vi "LET Output v2.vi"() -> ()   [LabVIEW 2010]
doc: "Cont(inuous) Acq(uire) & Chart (hw timed) demonstrates the hardware timed, non-buffered technique of data acquisition. The scan clock on the board controls acquisition timing. Acquired scans are read directly from the device's FIFO using AI Single Scan. \n\nThe acquisition is configured with no buffer, and the on-board scan clock started at the selected scan rate. In the first loop iteration, the newest (most recent) scan is read from the FIFO. In each subsequent loop iteration AI Single Scan is called to read the oldest scan from the FIFO. Then if a scan is missed because the acquisition does not keep up, an error message will be displayed, and the acquisition stopped. Each scan is plotted on the chart after it is read. \n\nA common reason to use non-buffered acquisition is that some kind of processing needs to be done for each data point. You will probably want to add more functions to the diagram to customize this VI for your application. The acquisition rate you can achieve depends on how much processing and display the VI must do. This VI calls a subVI named My Single-Scan Processing. Add whatever processing you need to this subVI, or replace it with one of your own. The data processing subVI also demonstrates how to use error clusters in your own subVIs, so they can be included in the error data flow chain.\n\nBefore running this VI, set the values of the controls on the front panel. Select Show Help Window from the Help menu to see a description of each control. If the values you select for all the controls are values you will usually use, select Make Current Values Default from the Operate menu and save the VI. Or, you may save individual control's default values by popping up on the control, selecting Data Operations, then selecting Make Current Value Default, and saving the VI."
uses:
  <instrlib>/agilent_b2900_series/Agilent B2900 Series/Public/Configure/Measurement/Configure Measurement (Current).vi
  <instrlib>/agilent_b2900_series/Agilent B2900 Series/Public/Configure/Measurement/Configure Measurement (Voltage).vi
  <vilib>/Analysis/Matrix/Numeric/Conversions/Matrix To Array - RM.vi
  <vilib>/Utility/file.llb/Write To Spreadsheet File (DBL).vi
  <instrlib>/agilent_b2900_series/Agilent B2900 Series/Agilent B2900 Series.lvlib
  <vilib>/Analysis/Matrix/NI_Matrix.lvlib
panel:
  out "Real 2D Array":dbl[][](array[numeric])
  out "data matrix":dbl[][](array[numeric])
  out "Igs array 2":dbl[][](array[numeric])
  out "Vgs array 2":dbl[][](array[numeric])
  out "Vds array 2":dbl[][](array[numeric])
  out "Corrected PD current array 2":dbl[][](array[numeric])
  out "Ids array 2":dbl[][](array[numeric])
  out "corrected PD current array":dbl[](array[numeric])
  out "Vds array":dbl[](array[numeric])
  out "Ids array":dbl[](array[numeric])
  out "Vgs array":dbl[](array[numeric])
  out "Igs array":dbl[](array[numeric])
  in  "Tab Control":T1(tab)
  in  "keithley address":string="GPIB0::20::INSTR"
  in  "agilent address":refnum<visa-resource-name>="GPIB0::23::INSTR"
  in  "Initial Vds (V)\n(100 scans/sec)":sgl caption="Initial Vds (V)" format="%.2f"
  in  "Vds step (V)":sgl=1.0 format="%.2f"
  in  "Vds delay time":sgl=10.0 caption="Vds delay time (ms)" format="%.2f"
  in  "Vds delay after first value (ms)":sgl=10.0 format="%.2f"
  in  "Final Vds(V)":sgl=60.0 format="%.2f"
  in  "light emission ON/OFF":bool=TRUE
  in  "Vgs step (V)":sgl=20.0 format="%.2f"
  in  "Final Vgs (V)":sgl=60.0 format="%.2f"
  in  "Initial Vgs (V)":sgl format="%.2f"
  in  "Vgs hold time (ms)":i32=10
  in  "Compliance Voltage (channel 2)":dbl=60.0
  in  "Compliance Current (channel 1)":dbl=0.001
  in  "Compliance Voltage (channel 1)":dbl=60.0
  in  "Compliance Current (channel 2)":dbl=0.0001
  in  "keithley compliance limit":dbl(ring)=0.025 items=["25uA"=2.5e-05, "250uA"=0.00025, "2.5mA"=0.0025, "25mA"=0.025]
  in  "Loop":bool=TRUE
  in  "keithley current resolution":dbl=0.0001 format="%^.2e"
  in  "Current Auto Range Mode (0: Normal)":i32(ring) items=["Normal", "Resolution", "Speed"]
  in  "Voltage Auto Range Mode (0: Normal)":i32(ring) items=["Normal", "Resolution", "Speed"]
  in  "aperture time":dbl(ring)=-2.0 format="%.2f" items=["KE6485_VAL_RATE_FAST"=-1.0, "KE6485_VAL_RATE_MEDIUM"=-2.0, "KE6485_VAL_RATE_SLOW"=-3.0]
  in  "Auto Current NPLC (F: Disable)":bool
  in  "Current NPLC (0.1)":dbl=0.1
  in  "Auto Voltage NPLC(F: Disable)":bool
  in  "Voltage NPLC (0.1 PLC)":dbl=0.1
  out "Current Scan":cluster{dbl[], dbl[]}(graph)
  out "Applied Vds":sgl caption="current VDS (V)" format="%.2f"
  out "Applied Vgs":sgl caption="current VDS (V)" format="%.2f"
  out "Measured Ids":dbl format="%.2e"
  out "Measured Vds":dbl
  out "corrected PD current":dbl format="%^.2e"
  out "dark PD current (A)":dbl format="%^.2e"
  out "PD current":dbl format="%^.2e"
  out "Measured Igs":dbl
  out "Measured Vgs":dbl
  out "channel 2 status":bool
  out "channel 1 status":bool
  out "Current Scan 2":cluster{dbl[], dbl[]}(graph) caption="Current Scan"
  out "half  points":sgl
  out "Vds points":sgl
  out "Vgs points":sgl
  out "?":cluster{dbl[], dbl[]}[](graph)
  out "?":cluster{dbl[], dbl[]}[](graph)
  in  "error in keithley":errorcluster
  out "keithley address out":refnum<k15>
  out "error out keithley":errorcluster
  out "error out agilent":errorcluster
  out "Agilent address out":refnum<visa-resource-name>
  # "FET output v2"
  # "Drain-Source Setting"
  # "Gate Setting"
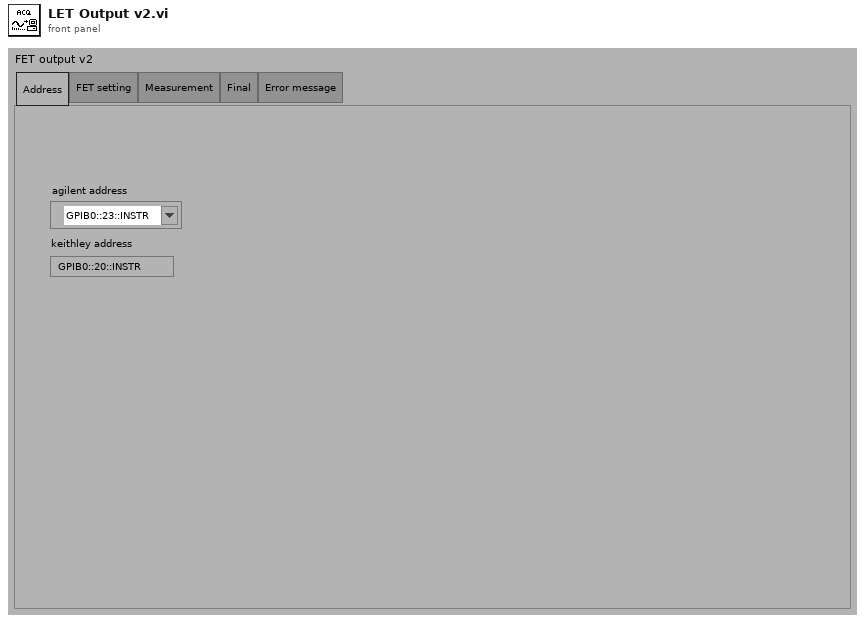
[diagram p1: front panel]
types:
  T1 = enum32{"Address", "FET setting", "Measurement", "Final", "Error message"}
  T2 = typedef "NI_Matrix.lvlib/RealMatrix.ctl" = dbl[][]
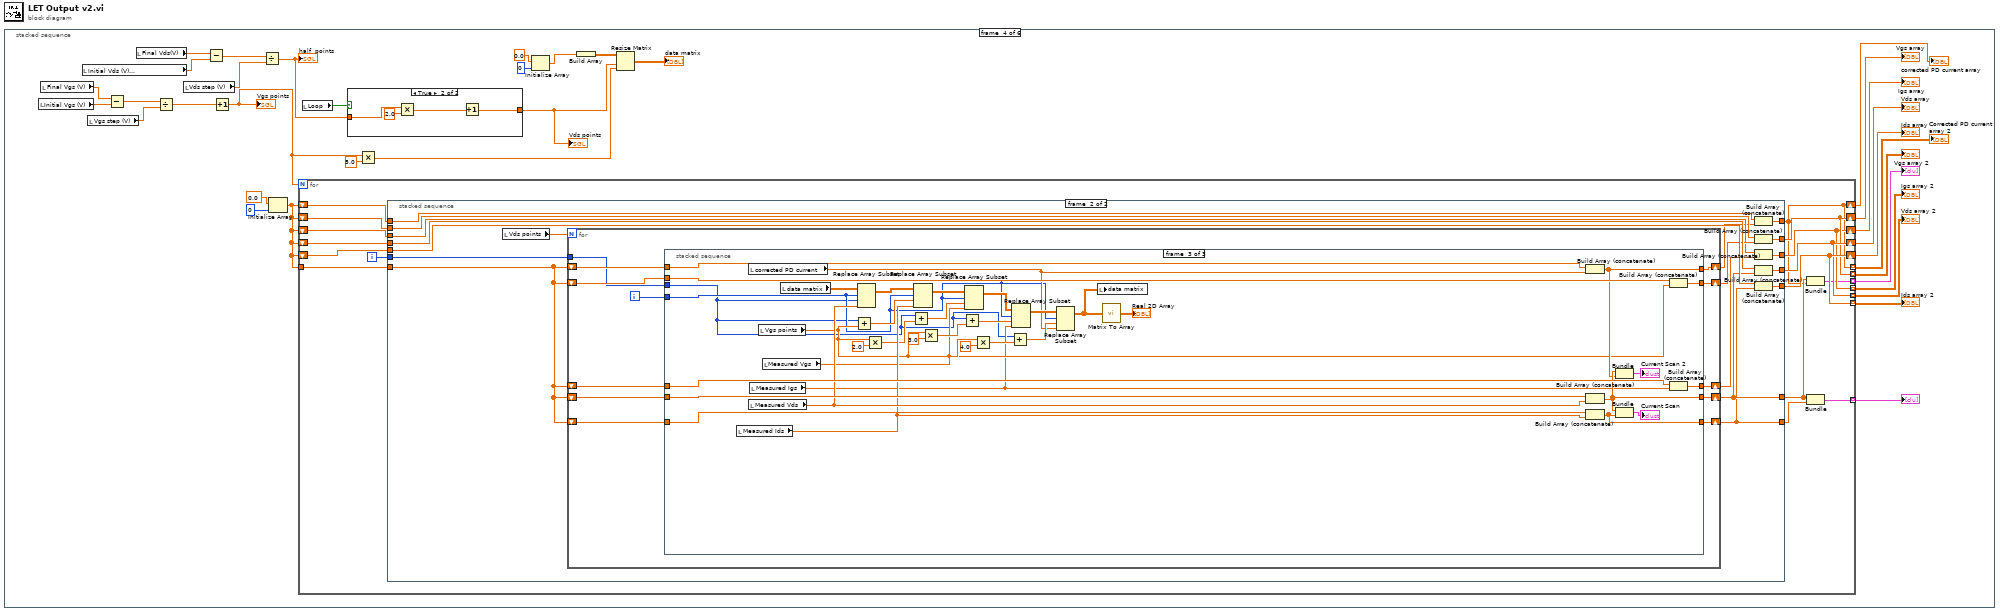
[diagram p0: block diagram]
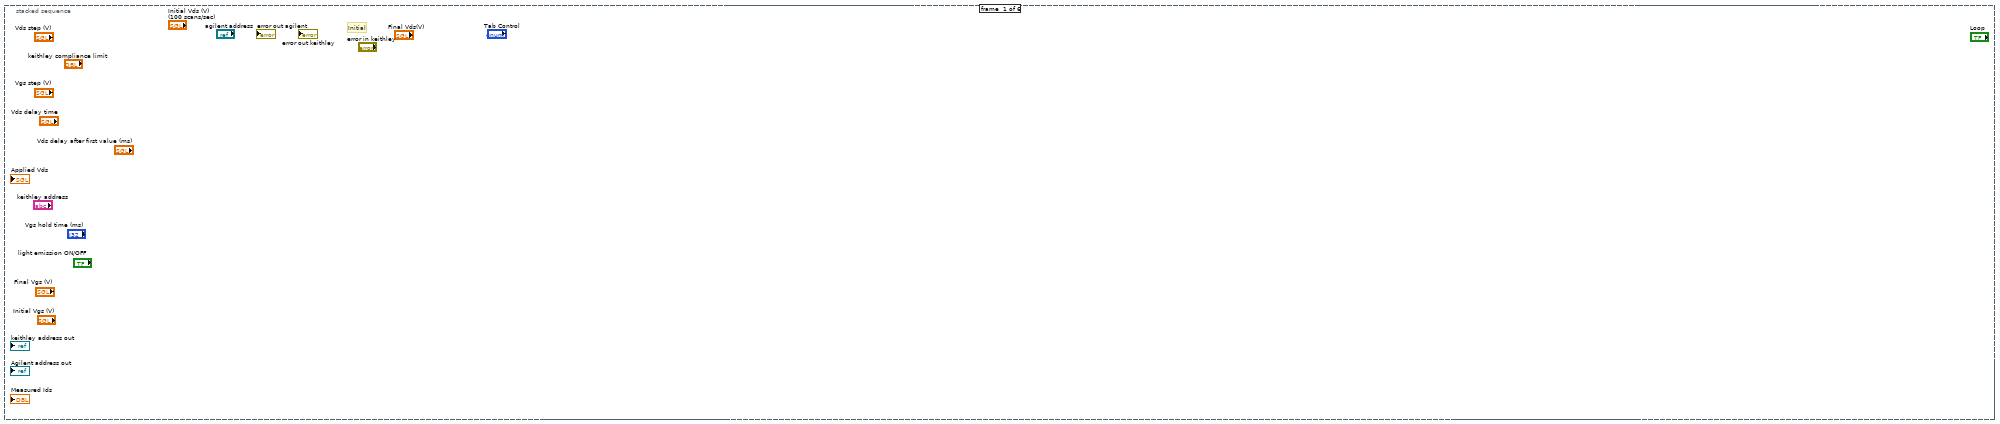
[diagram p2: hidden frame]
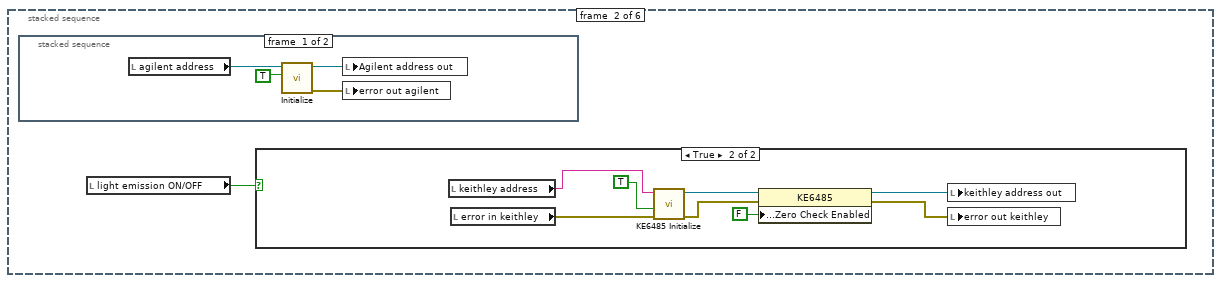
[diagram p3: hidden frame]
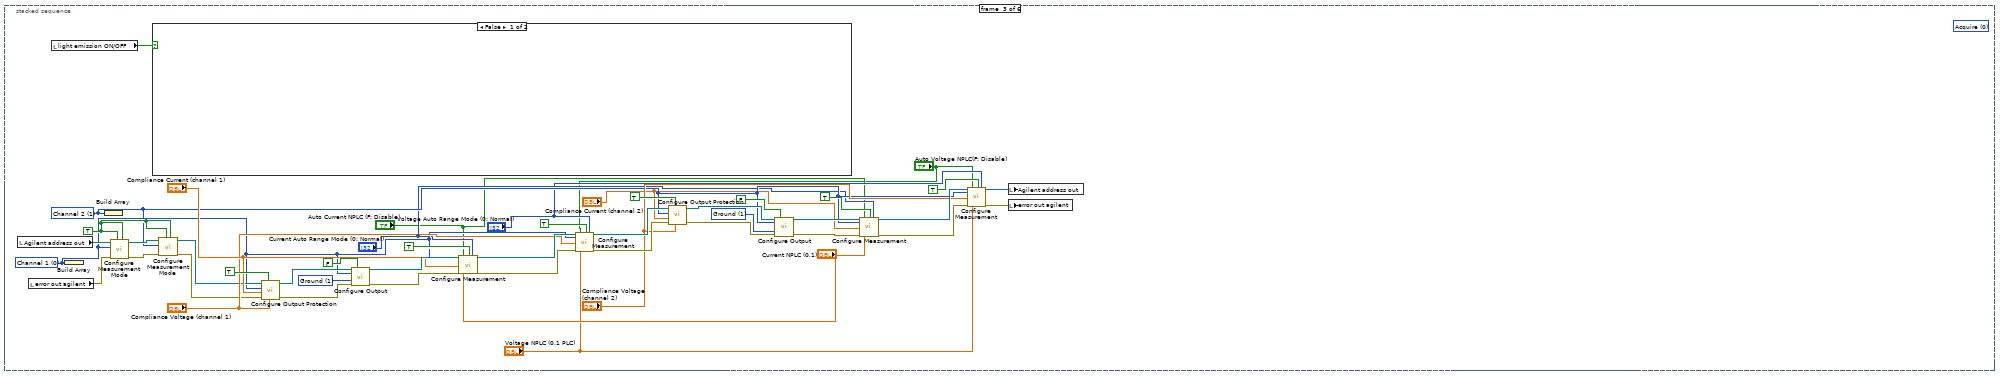
[diagram p6: hidden frame]
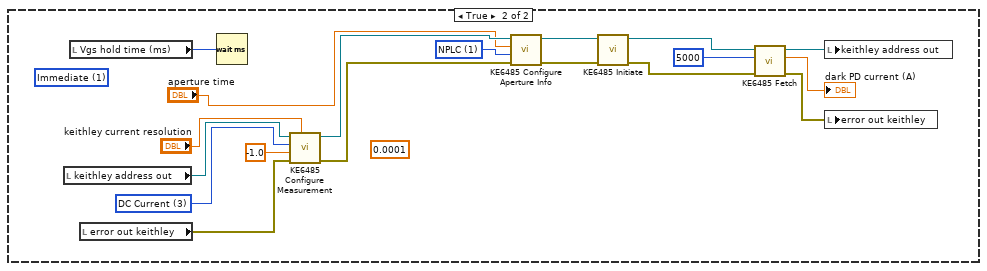
[diagram p7: hidden frame]
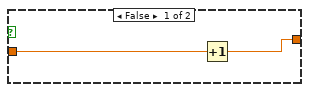
[diagram p8: hidden frame]
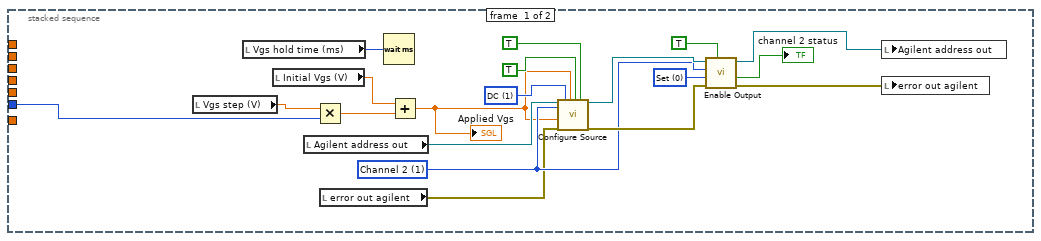
[diagram p9: hidden frame]
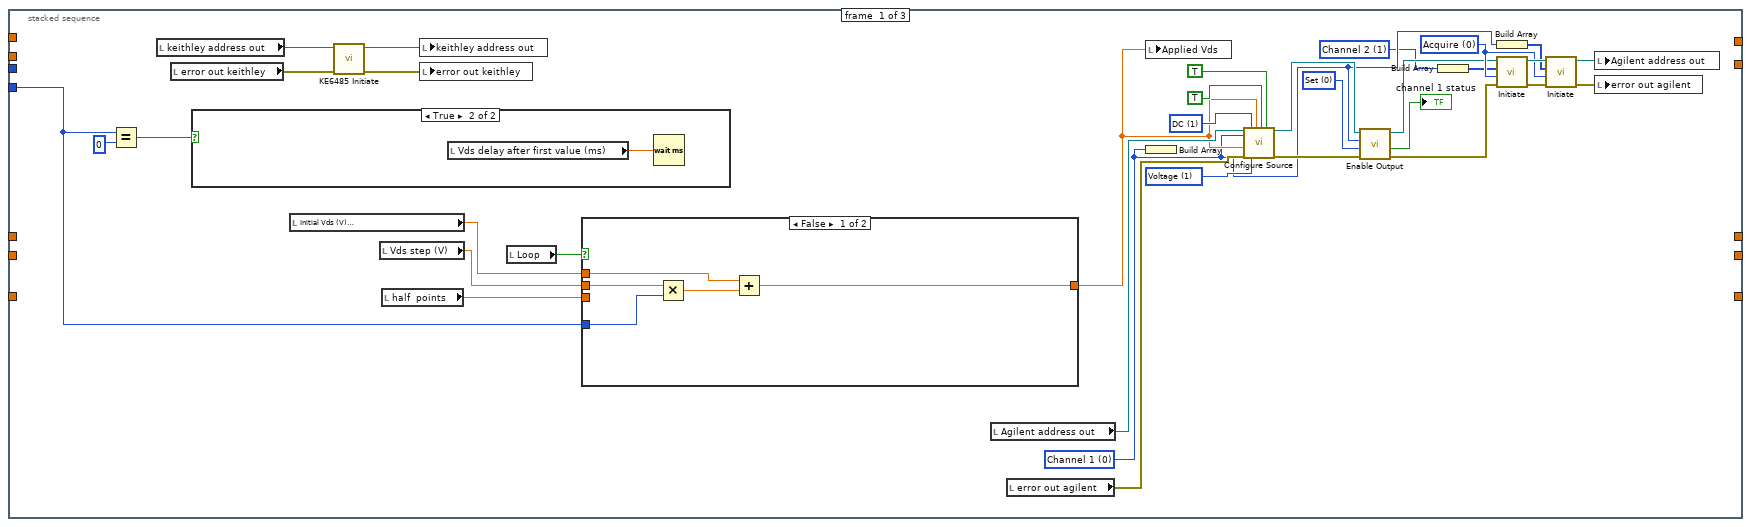
[diagram p10: hidden frame]
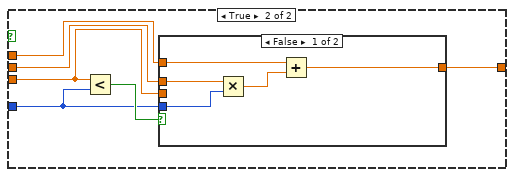
[diagram p11: hidden frame]
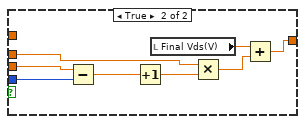
[diagram p12: hidden frame]
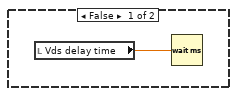
[diagram p13: hidden frame]
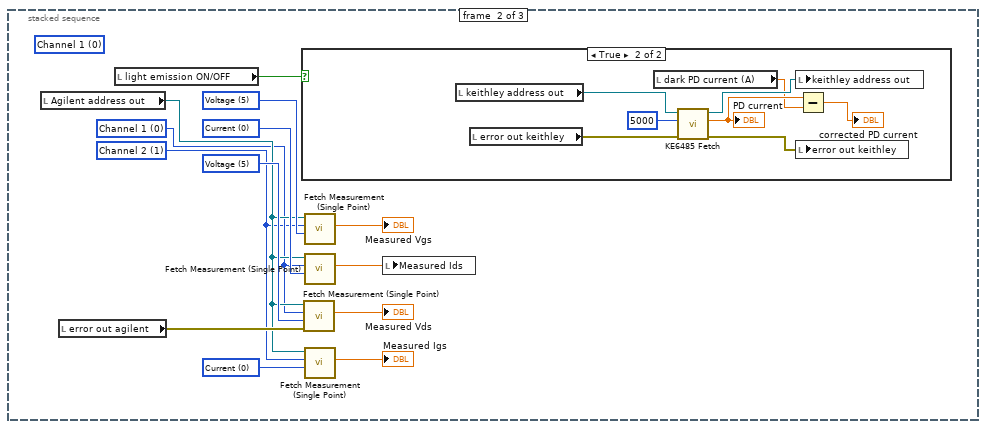
[diagram p14: hidden frame]
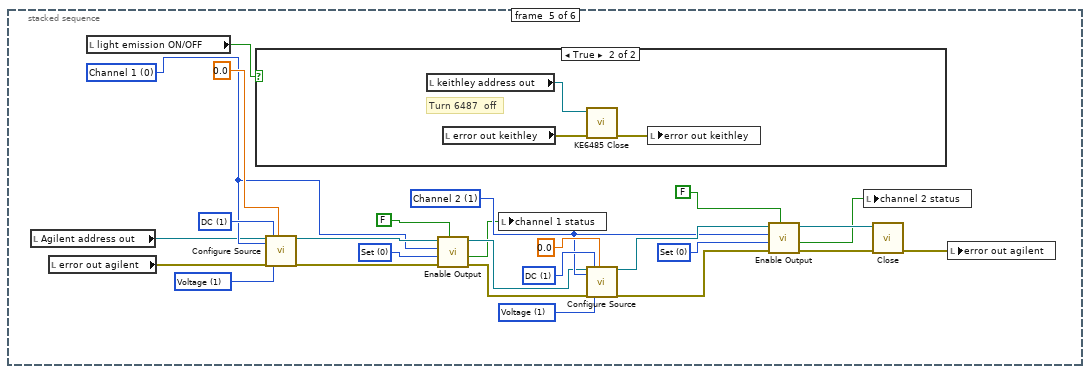
[diagram p16: hidden frame]
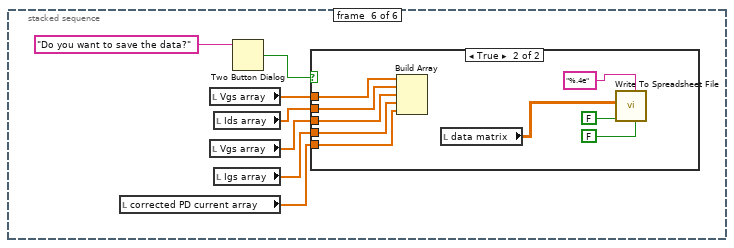
[diagram p18: hidden frame]
diagram:
  n1 = stacked-sequence {
    frame #0 {
      # "Initial"
    }
    frame #1 {
      n2 = stacked-sequence {
        frame #0 {
          n3 = local read "agilent address"() -> (w2:refnum<visa-resource-name>)
          n4 = call <instrlib>:"Initialize.vi"("ID Query (True)"=TRUE, "VISA resource name"=w2) -> ("error out"=w3:errorcluster, "VISA resource name out"=w4:refnum<visa-resource-name>)  [unwired: 8 in]
          n5 = local write "Agilent address out"(w4) -> ()
          n6 = local write "error out agilent"(w3) -> ()
        }
        frame #1 {
        }
      }
      n7 = local read "light emission ON/OFF"() -> (w1:bool)
      n8 = case shown="True" w1 {
        frame False {
        }
        frame True {
          n9 = local read "keithley address"() -> (w12:string)
          n10 = local read "error in keithley"() -> (w13:errorcluster)
          n11 = call <instrlib>:"KE6485 Initialize.vi"("error in (no error)"=w13, "reset device"=TRUE, "resource name"=w12) -> ("error out"=w10:errorcluster, "instrument handle out"=w9:refnum<k15>)  [unwired: 1 in, 6 out]
          n12 = property class="KE6485"(reference=w9, error in=w10, "System Settings:Zero Check Enabled"=FALSE) -> (reference out=w8:refnum<k15>, error out=w7:errorcluster)
          n13 = local write "keithley address out"(w8) -> ()
          n14 = local write "error out keithley"(w7) -> ()
        }
      }
    }
    frame #2 {
      (unwired) 0 items=["Acquire", "Transient", "Both"] ("Device Action (2: Both)")
      w30 = TRUE ("Enable Voltage Measurement (T: Enable)")
      w42 = 1 items=["Float", "Ground"] ("Low Terminal State (1: Ground)")
      w22 = 1 items=["Channel 1", "Channel 2"] ("Channel (0: Channel 1)")
      w52 = 1 items=["Float", "Ground"] ("Low Terminal State (1: Ground)")
      w23 = 0 items=["Channel 1", "Channel 2"] ("Channel (0: Channel 1)")
      n15 = local read "Agilent address out"() -> (w25:refnum<visa-resource-name>)
      n16 = local read "error out agilent"() -> (w27:errorcluster)
      n17 = local read "light emission ON/OFF"() -> (w59:bool)
      n18 = Build Array(w23) -> ()  [unwired: 1 out]
      n19 = Build Array(w22) -> ()  [unwired: 1 out]
      n20 = call <instrlib>:"Configure Measurement Mode.vi"("Enable Current Measurement (T: Enable)"=w30, "Enable Voltage Measurement (T: Enable)"=w30, "error in (no error)"=w27, "Channel (0: Channel 1)"=w23, "VISA resource name"=w25) -> ("error out"=w28:errorcluster, "VISA resource name out"=w29:refnum<visa-resource-name>)  [unwired: 5 in]
      n21 = case shown="False" w59 {
        frame False {
        }
        frame True {
          w65 = 1 items=["NPLC"=1] ("aperture time unit")
          (unwired) 0.0001 ("resolution (absolute)")
          (unwired) 1 items=["Immediate"=1, "Interval"=10, "Trigger Link 1"=1001, "Trigger Link 2"=1002, "Trigger Link 3"=1003, "Trigger Link 4"=1004, "Trigger Link 5"=1005, "Trigger Link 6"=1006] ("sample trigger")
          w75 = 3 items=["DC Volts"=1, "DC Current"=3, "2 Wire Resistance"=5, "Charge"=1004] ("measurement function")
          n22 = local read "keithley address out"() -> (w70:refnum<k15>)
          n23 = local read "Vgs hold time (ms)"() -> (w77:i32)
          n24 = local read "error out keithley"() -> (w69:errorcluster)
          n25 = Wait (ms)(milliseconds to wait=w77) -> ()  [unwired: 1 out]
          n26 = call <instrlib>:"KE6485 Configure Measurement.vi"("resolution (absolute)"="keithley current resolution", "error in (no error)"=w69, "range"=-1.0, "measurement function"=w75, "instrument handle"=w70) -> ("error out"=w64:errorcluster, "instrument handle out"=w63:refnum<k15>)  [unwired: 5 in]
          n27 = call <instrlib>:"KE6485 Configure Aperture Info.vi"("error in (no error)"=w64, "aperture time unit"=w65, "aperture time"="aperture time", "instrument handle"=w63) -> ("error out"=w61:errorcluster, "instrument handle out"=w62:refnum<k15>)  [unwired: 6 in]
          n28 = call <instrlib>:"KE6485 Initiate.vi"("error in (no error)"=w61, "instrument handle"=w62) -> ("error out"=w67:errorcluster, "instrument handle out"=w68:refnum<k15>)  [unwired: 8 in]
          n29 = call <instrlib>:"KE6485 Fetch.vi"("error in (no error)"=w67, "maximum time (ms)"=5000, "instrument handle"=w68) -> ("error out"=w72:errorcluster, "reading"=→"dark PD current (A)":dbl, "instrument handle out"=w71:refnum<k15>)  [unwired: 6 in]
          n30 = local write "keithley address out"(w71) -> ()
          n31 = local write "error out keithley"(w72) -> ()
        }
      }
      n32 = call <instrlib>:"Configure Measurement Mode.vi"("Enable Current Measurement (T: Enable)"=w30, "Enable Voltage Measurement (T: Enable)"=w30, "error in (no error)"=w28, "Channel (0: Channel 1)"=w22, "VISA resource name"=w29) -> ("error out"=w26:errorcluster, "VISA resource name out"=w24:refnum<visa-resource-name>)  [unwired: 5 in]
      n33 = call <instrlib>:"Configure Output Protection.vi"("Compliance Voltage (2 V)"="Compliance Voltage (channel 1)", "Enable Output Protection (T: Enable)"=TRUE, "error in (no error)"=w26, "Compliance Current (0.0001 A)"="Compliance Current (channel 1)", "Channel (0: Channel 1)"=w23, "VISA resource name"=w24) -> ("error out"=w54:errorcluster, "VISA resource name out"=w53:refnum<visa-resource-name>)  [unwired: 4 in]
      n34 = call <instrlib>:"Configure Output.vi"("VISA resource name"=w53, "Auto Output-Off (F: Disable)"=FALSE, "Channel (0: Channel 1)"=w23, "Low Terminal State (1: Ground)"=w52, "error in (no error)"=w54) -> ("VISA resource name out"=w50:refnum<visa-resource-name>, "error out"=w51:errorcluster)  [unwired: 9 in]
      n35 = call-poly <instrlib>:"Configure Measurement.vi"("VISA resource name"=w50, "Channel (0: Channel 1)"=w23, "Current Range (0.0001 A)"="Compliance Current (channel 1)", "error in (no error)"=w51, "Auto Current NPLC (F: Disable)"="Auto Current NPLC (F: Disable)", "Current NPLC (0.1)"="Current NPLC (0.1)", "Current Auto Range (T: Enable)"=TRUE, "Current Auto Range Mode (0: Normal)"="Current Auto Range Mode (0: Normal)") -> ("VISA resource name out"=w58:refnum<visa-resource-name>, "error out"=w57:errorcluster)  [unwired: 10 in]
      n36 = call-poly <instrlib>:"Configure Measurement.vi"("VISA resource name"=w58, "Channel (0: Channel 1)"=w23, "Voltage Range (2 V)"="Compliance Voltage (channel 1)", "error in (no error)"=w57, "Auto Voltage NPLC(F: Disable)"="Auto Voltage NPLC(F: Disable)", "Voltage NPLC (0.1 PLC)"="Voltage NPLC (0.1 PLC)", "Voltage Auto Range (T: Enable)"=TRUE, "Voltage Auto Range Mode (0: Normal)"="Voltage Auto Range Mode (0: Normal)") -> ("VISA resource name out"=w38:refnum<visa-resource-name>, "error out"=w37:errorcluster)  [unwired: 10 in]
      n37 = call <instrlib>:"Configure Output Protection.vi"("Compliance Voltage (2 V)"="Compliance Voltage (channel 2)", "Enable Output Protection (T: Enable)"=TRUE, "error in (no error)"=w37, "Compliance Current (0.0001 A)"="Compliance Current (channel 2)", "Channel (0: Channel 1)"=w22, "VISA resource name"=w38) -> ("error out"=w44:errorcluster, "VISA resource name out"=w43:refnum<visa-resource-name>)  [unwired: 4 in]
      n38 = call <instrlib>:"Configure Output.vi"("VISA resource name"=w43, "Auto Output-Off (F: Disable)"=FALSE, "Channel (0: Channel 1)"=w22, "Low Terminal State (1: Ground)"=w42, "error in (no error)"=w44) -> ("VISA resource name out"=w40:refnum<visa-resource-name>, "error out"=w41:errorcluster)  [unwired: 9 in]
      n39 = call-poly <instrlib>:"Configure Measurement.vi"("VISA resource name"=w40, "Channel (0: Channel 1)"=w22, "Current Range (0.0001 A)"="Compliance Current (channel 2)", "error in (no error)"=w41, "Auto Current NPLC (F: Disable)"="Auto Current NPLC (F: Disable)", "Current NPLC (0.1)"="Current NPLC (0.1)", "Current Auto Range (T: Enable)"=TRUE, "Current Auto Range Mode (0: Normal)"="Current Auto Range Mode (0: Normal)") -> ("VISA resource name out"=w48:refnum<visa-resource-name>, "error out"=w47:errorcluster)  [unwired: 10 in]
      n40 = call-poly <instrlib>:"Configure Measurement.vi"("VISA resource name"=w48, "Channel (0: Channel 1)"=w22, "Voltage Range (2 V)"="Compliance Voltage (channel 2)", "error in (no error)"=w47, "Auto Voltage NPLC(F: Disable)"="Auto Voltage NPLC(F: Disable)", "Voltage NPLC (0.1 PLC)"="Voltage NPLC (0.1 PLC)", "Voltage Auto Range (T: Enable)"=TRUE, "Voltage Auto Range Mode (0: Normal)"="Voltage Auto Range Mode (0: Normal)") -> ("VISA resource name out"=w21:refnum<visa-resource-name>, "error out"=w20:errorcluster)  [unwired: 10 in]
      n41 = local write "Agilent address out"(w21) -> ()
      n42 = local write "error out agilent"(w20) -> ()
    }
    frame #3 {
      n43 = local read "Initial Vgs (V)"() -> (w101:sgl)
      n44 = local read "Final Vgs (V)"() -> (w100:sgl)
      n45 = local read "Initial Vds (V)\n(100 scans/sec)"() -> (w104:sgl)
      n46 = local read "Vgs step (V)"() -> (w102:sgl)
      n47 = Subtract(x=w100, y=w101) -> (x-y=w98:sgl)
      n48 = local read "Final Vds(V)"() -> (w103:sgl)
      n49 = Divide(x=w98, y=w102) -> (x/y=w99:sgl)
      n50 = local read "Vds step (V)"() -> (w105:sgl)
      n51 = Subtract(x=w103, y=w104) -> (x-y=w112:sgl)
      n52 = Increment(x=w99) -> (x+1=w84:sgl)
      "Vgs points" <- w84
      n53 = Divide(x=w112, y=w105) -> (x/y=w96:sgl)
      "half  points" <- w96
      n54 = Initialize Array(0.0, 0) -> (w93:dbl[])
      n55 = for {
        N: w84 -> [_]
        shift-right: [w125] -> w108
        shift-left: w93 -> [w133]
        shift-right: [w126] -> w109
        shift-left: w93 -> [w132]
        shift-right: [w123] -> w107
        shift-left: w93 -> [w131]
        tunnel: [w130] -> w106 mode=indexing
        shift-right: [w122] -> w95
        shift-left: w93 -> [w129]
        shift-right: [w120] -> w94
        shift-left: w93 -> [w128]
        tunnel: w93 -> [w127]
        tunnel: [w126] -> w92 mode=indexing
        tunnel: [w120] -> w91 mode=indexing
        tunnel: [w125] -> w90 mode=indexing
        tunnel: [w123] -> w89 mode=indexing
        tunnel: [w122] -> w88 mode=indexing
        tunnel: [w119] -> w87 mode=indexing
        i -> [w134]
        n56 = stacked-sequence {
          tunnel: w134 -> [w149 w154]
          tunnel: w133 -> [_ w171]
          tunnel: w132 -> [_ w170]
          tunnel: [_ w165] -> w125
          tunnel: [_ w169] -> w126
          tunnel: w131 -> [_ w167]
          tunnel: [_ w166] -> w123
          tunnel: [_ w164] -> w121
          tunnel: [_ w163] -> w124
          tunnel: w129 -> [_ w162]
          tunnel: [_ w161] -> w122
          tunnel: [_ w159] -> w120
          tunnel: w128 -> [_ w157]
          tunnel: w127 -> [_ w155]
          frame #0 {
            w142 = 0 items=["Set", "Get"] ("Operation (0: Set)")
            w143 = 1 items=["Channel 1", "Channel 2"] ("Channel (0: Channel 1)")
            w146 = 1 items=["Pulse", "DC"] ("Source Shape (1: DC)")
            n57 = local read "Vgs step (V)"() -> (w153:sgl)
            n58 = local read "Vgs hold time (ms)"() -> (w151:i32)
            n59 = local read "Initial Vgs (V)"() -> (w152:sgl)
            n60 = local read "Agilent address out"() -> (w139:refnum<visa-resource-name>)
            n61 = Multiply(x=w153, y=w149) -> (x*y=w150:sgl)
            n62 = local read "error out agilent"() -> (w138:errorcluster)
            n63 = Wait (ms)(milliseconds to wait=w151) -> ()  [unwired: 1 out]
            n64 = Add(x=w152, y=w150) -> (x+y=w135:sgl)
            "Applied Vgs" <- w135
            n65 = call <instrlib>:"Configure Source.vi"("VISA resource name"=w139, "Channel (0: Channel 1)"=w143, "Source Range (2)"=w135, "error in (no error)"=w138, "Source Shape (1: DC)"=w146, "Output Level (0)"=w135, "Source Auto Range (T: Enable)"=TRUE, "Enable Continuous Output (T: Enable)"=TRUE) -> ("VISA resource name out"=w148:refnum<visa-resource-name>, "error out"=w147:errorcluster)  [unwired: 10 in]
            n66 = call <instrlib>:"Enable Output.vi"("Enable Output (T: Enable)"=TRUE, "error in (no error)"=w147, "Operation (0: Set)"=w142, "Channel (0: Channel 1)"=w143, "VISA resource name"=w148) -> ("error out"=w137:errorcluster, "Output Enabled?"=→"channel 2 status":bool, "VISA resource name out"=w136:refnum<visa-resource-name>)  [unwired: 4 in]
            n67 = local write "Agilent address out"(w136) -> ()
            n68 = local write "error out agilent"(w137) -> ()
          }
          frame #1 {
            n69 = local read "Vds points"() -> (w156:sgl)
            n70 = for {
              N: w156 -> [_]
              shift-right: [w174] -> w163
              shift-left: w155 -> [w173]
              shift-right: [w176] -> w164
              shift-left: w155 -> [w175]
              shift-right: [w180] -> w168
              shift-left: w155 -> [w179]
              shift-right: [w178] -> w160
              shift-left: w155 -> [w177]
              shift-right: [w181] -> w158
              shift-left: w155 -> [w182]
              tunnel: w154 -> [w172]
              i -> [w183]
              n71 = stacked-sequence {
                tunnel: w183 -> [w203 _ w265]
                tunnel: w182 -> [_ _ w300]
                tunnel: [_ _ w289] -> w181
                tunnel: [_ _ w299] -> w180
                tunnel: w179 -> [_ _ w298]
                tunnel: [_ _ w297] -> w178
                tunnel: w177 -> [_ _ w296]
                tunnel: [_ _ w290] -> w176
                tunnel: w175 -> [_ _ w294]
                tunnel: [_ _ w292] -> w174
                tunnel: w173 -> [_ _ w293]
                tunnel: w172 -> [_ _ w264]
                frame #0 {
                  w196 = 0 items=["Acquire", "Transient", "Both"] ("Device Action (2: Both)")
                  w188 = 1 items=["Channel 1", "Channel 2"] ("Channel (0: Channel 1)")
                  w205 = 1 items=["Current", "Voltage"] ("Source Mode (1: Voltage)")
                  w208 = 1 items=["Pulse", "DC"] ("Source Shape (1: DC)")
                  w189 = 0 items=["Channel 1", "Channel 2"] ("Channel (0: Channel 1)")
                  w212 = 0 items=["Set", "Get"] ("Operation (0: Set)")
                  n72 = Equal?(x=w203, y=0) -> (x = y?=w215:bool)
                  n73 = local read "keithley address out"() -> (w185:refnum<k15>)
                  n74 = local read "error out keithley"() -> (w184:errorcluster)
                  n75 = case shown="True" w215 {
                    frame False {
                      n76 = local read "Vds delay time"() -> (w241:sgl)
                      n77 = Wait (ms)(milliseconds to wait=w241) -> ()  [unwired: 1 out]
                    }
                    frame True {
                      n78 = local read "Vds delay after first value (ms)"() -> (w242:sgl)
                      n79 = Wait (ms)(milliseconds to wait=w242) -> ()  [unwired: 1 out]
                    }
                  }
                  n80 = local read "Initial Vds (V)\n(100 scans/sec)"() -> (w204:sgl)
                  n81 = call <instrlib>:"KE6485 Initiate.vi"("error in (no error)"=w184, "instrument handle"=w185) -> ("error out"=w187:errorcluster, "instrument handle out"=w186:refnum<k15>)  [unwired: 8 in]
                  n82 = local read "Vds step (V)"() -> (w202:sgl)
                  n83 = local read "half  points"() -> (w200:sgl)
                  n84 = local write "keithley address out"(w186) -> ()
                  n85 = local write "error out keithley"(w187) -> ()
                  n86 = local read "Loop"() -> (w201:bool)
                  n87 = case shown="False" w201 {
                    tunnel: [w220 w226] -> w199
                    tunnel: w203 -> [w219 w223]
                    tunnel: w204 -> [w218 w225]
                    tunnel: w202 -> [w217 w224]
                    tunnel: w200 -> [_ w222]
                    frame False {
                      n88 = Multiply(x=w217, y=w219) -> (x*y=w221:sgl)
                      n89 = Add(x=w218, y=w221) -> (x+y=w220:sgl)
                    }
                    frame True {
                      n90 = Less?(x=w222, y=w223) -> (x < y?=w227:bool)
                      n91 = case shown="False" w227 {
                        tunnel: [w231 w240] -> w226
                        tunnel: w225 -> [w230 _]
                        tunnel: w223 -> [w229 w237]
                        tunnel: w224 -> [w228 w238]
                        tunnel: w222 -> [_ w236]
                        frame False {
                          n92 = Multiply(x=w228, y=w229) -> (x*y=w232:sgl)
                          n93 = Add(x=w230, y=w232) -> (x+y=w231:sgl)
                        }
                        frame True {
                          n94 = Subtract(x=w236, y=w237) -> (x-y=w234:sgl)
                          n95 = Increment(x=w234) -> (x+1=w233:sgl)
                          n96 = local read "Final Vds(V)"() -> (w235:sgl)
                          n97 = Multiply(x=w238, y=w233) -> (x*y=w239:sgl)
                          n98 = Add(x=w235, y=w239) -> (x+y=w240:sgl)
                        }
                      }
                    }
                  }
                  n99 = local read "Agilent address out"() -> (w210:refnum<visa-resource-name>)
                  n100 = local read "error out agilent"() -> (w209:errorcluster)
                  n101 = local write "Applied Vds"(w199) -> ()
                  n102 = Build Array(w189) -> ()  [unwired: 1 out]
                  n103 = call <instrlib>:"Configure Source.vi"("VISA resource name"=w210, "Channel (0: Channel 1)"=w189, "Source Range (2)"=w199, "error in (no error)"=w209, "Source Shape (1: DC)"=w208, "Source Mode (1: Voltage)"=w205, "Output Level (0)"=w199, "Source Auto Range (T: Enable)"=TRUE, "Enable Continuous Output (T: Enable)"=TRUE) -> ("VISA resource name out"=w214:refnum<visa-resource-name>, "error out"=w213:errorcluster)  [unwired: 9 in]
                  n104 = call <instrlib>:"Enable Output.vi"("error in (no error)"=w213, "Operation (0: Set)"=w212, "Channel (0: Channel 1)"=w189, "VISA resource name"=w214) -> ("error out"=w192:errorcluster, "Output Enabled?"=→"channel 1 status":bool, "VISA resource name out"=w193:refnum<visa-resource-name>)  [unwired: 5 in]
                  n105 = Build Array(w188) -> (w195:i32[])
                  n106 = Build Array(w189) -> (w194:i32[])
                  n107 = call <instrlib>:"Initiate.vi"("error in (no error)"=w192, "Device Action (2: Both)"=w196, "Channel List ({Channel1})"=w195, "VISA resource name"=w193) -> ("error out"=w198:errorcluster, "VISA resource name out"=w197:refnum<visa-resource-name>)  [unwired: 6 in]
                  n108 = call <instrlib>:"Initiate.vi"("error in (no error)"=w198, "Device Action (2: Both)"=w196, "Channel List ({Channel1})"=w194, "VISA resource name"=w197) -> ("error out"=w191:errorcluster, "VISA resource name out"=w190:refnum<visa-resource-name>)  [unwired: 6 in]
                  n109 = local write "Agilent address out"(w190) -> ()
                  n110 = local write "error out agilent"(w191) -> ()
                }
                frame #1 {
                  w244 = 1 items=["Channel 1", "Channel 2"] ("Channel (0: Channel 1)")
                  w245 = 0 items=["Channel 1", "Channel 2"] ("Channel (0: Channel 1)")
                  w250 = 0 items=["Current", "Resistance", "Source Output Setting", "Status", "Time", "Voltage"] ("Data Mode (5: Voltage)")
                  w251 = 5 items=["Current", "Resistance", "Source Output Setting", "Status", "Time", "Voltage"] ("Data Mode (5: Voltage)")
                  w253 = 0 items=["Current", "Resistance", "Source Output Setting", "Status", "Time", "Voltage"] ("Data Mode (5: Voltage)")
                  (unwired) 0 items=["Channel 1", "Channel 2"] ("Channel (0: Channel 1)")
                  w255 = 5 items=["Current", "Resistance", "Source Output Setting", "Status", "Time", "Voltage"] ("Data Mode (5: Voltage)")
                  n111 = local read "Agilent address out"() -> (w246:refnum<visa-resource-name>)
                  n112 = local read "error out agilent"() -> (w247:errorcluster)
                  n113 = local read "light emission ON/OFF"() -> (w243:bool)
                  n114 = case shown="True" w243 {
                    frame False {
                    }
                    frame True {
                      n115 = local read "keithley address out"() -> (w257:refnum<k15>)
                      n116 = local read "error out keithley"() -> (w256:errorcluster)
                      n117 = local read "dark PD current (A)"() -> (w258:dbl)
                      n118 = call <instrlib>:"KE6485 Fetch.vi"("error in (no error)"=w256, "maximum time (ms)"=5000, "instrument handle"=w257) -> ("error out"=w262:errorcluster, "reading"=w259:dbl, "instrument handle out"=w261:refnum<k15>)  [unwired: 6 in]
                      "PD current" <- w259
                      n119 = local write "keithley address out"(w261) -> ()
                      n120 = local write "error out keithley"(w262) -> ()
                      n121 = Subtract(x=w259, y=w258) -> (x-y=→"corrected PD current":dbl)
                    }
                  }
                  n122 = call <instrlib>:"Fetch Measurement (Single Point).vi"("error in (no error)"=w247, "Data Mode (5: Voltage)"=w255, "Channel (0: Channel 1)"=w245, "VISA resource name"=w246) -> ("Measurement"=→"Measured Vds":dbl)  [unwired: 5 in, 2 out]
                  n123 = call <instrlib>:"Fetch Measurement (Single Point).vi"("Data Mode (5: Voltage)"=w251, "Channel (0: Channel 1)"=w244, "VISA resource name"=w246) -> ("Measurement"=→"Measured Vgs":dbl)  [unwired: 6 in, 2 out]
                  n124 = call <instrlib>:"Fetch Measurement (Single Point).vi"("Data Mode (5: Voltage)"=w253, "Channel (0: Channel 1)"=w245, "VISA resource name"=w246) -> ("Measurement"=w252:dbl)  [unwired: 6 in, 2 out]
                  n125 = call <instrlib>:"Fetch Measurement (Single Point).vi"("Data Mode (5: Voltage)"=w250, "Channel (0: Channel 1)"=w244, "VISA resource name"=w246) -> ("Measurement"=→"Measured Igs":dbl)  [unwired: 6 in, 2 out]
                  n126 = local write "Measured Ids"(w252) -> ()
                }
                frame #2 {
                  n127 = local read "Measured Ids"() -> (w284:dbl)
                  n128 = local read "corrected PD current"() -> (w268:dbl)
                  n129 = local read "Measured Vds"() -> (w287:dbl)
                  n130 = local read "Measured Igs"() -> (w269:dbl)
                  n131 = local read "Vgs points"() -> (w271:sgl)
                  n132 = local read "Measured Vgs"() -> (w270:dbl)
                  n133 = local read "data matrix"() -> (w288:dbl[][])
                  n134 = Add(x=w264, y=w271) -> (x+y=w285:sgl)
                  n135 = Replace Array Subset(array=w288, new element=w287, index (row)=w265, index (col)=w264) -> (w286:T2)
                  n136 = Multiply(x=w271, y=sgl 2.0) -> (x*y=w281:sgl)
                  n137 = Add(x=w264, y=w281) -> (x+y=w282:sgl)
                  n138 = Replace Array Subset(array=w286, new element=w284, index (row)=w265, index (col)=w285) -> (w283:T2)
                  n139 = Multiply(x=w271, y=sgl 3.0) -> (x*y=w278:sgl)
                  n140 = Add(x=w264, y=w278) -> (x+y=w276:sgl)
                  n141 = Replace Array Subset(array=w283, new element=w270, index (row)=w265, index (col)=w282) -> (w279:T2)
                  n142 = Multiply(x=w271, y=sgl 4.0) -> (x*y=w274:sgl)
                  n143 = Add(x=w264, y=w274) -> (x+y=w272:sgl)
                  n144 = Replace Array Subset(array=w279, new element=w269, index (row)=w265, index (col)=w276) -> (w275:T2)
                  n145 = Replace Array Subset(array=w275, new element=w268, index (row)=w265, index (col)=w272) -> (w267:T2)
                  n146 = local write "data matrix"(w267) -> ()
                  n147 = call-poly <vilib>:"Matrix To Array.vi"("Real Matrix"=w267) -> ("Real 2D Array"=→"Real 2D Array":dbl[][])
                  n148 = Build Array (concatenate)(w300, w268) -> (w289:dbl[])
                  n149 = Build Array (concatenate)(w294, w287) -> (w290:dbl[])
                  n150 = Build Array (concatenate)(w293, w284) -> (w292:dbl[])
                  n151 = Bundle(w290, w289) -> (→"Current Scan 2":cluster{dbl[], dbl[]})  [unwired: 1 out]
                  n152 = Bundle(w290, w292) -> (→"Current Scan":cluster{dbl[], dbl[]})  [unwired: 1 out]
                  n153 = Build Array (concatenate)(w298, w270) -> (w299:dbl[])
                  n154 = Build Array (concatenate)(w296, w269) -> (w297:dbl[])
                }
              }
            }
            n155 = Build Array (concatenate)(w157, w158) -> (w159:dbl[])
            n156 = Build Array (concatenate)(w167, w168) -> (w166:dbl[])
            n157 = Build Array (concatenate)(w162, w160) -> (w161:dbl[])
            n158 = Build Array (concatenate)(w171, w164) -> (w165:dbl[])
            n159 = Build Array (concatenate)(w170, w163) -> (w169:dbl[])
          }
        }
        n160 = Bundle(w121, w120) -> (w119:cluster{dbl[], dbl[]})  [unwired: 1 out]
        n161 = Bundle(w121, w124) -> (w130:cluster{dbl[], dbl[]})  [unwired: 1 out]
      }
      "?" <- w106
      "Igs array" <- w95
      "Vgs array" <- w107
      "Ids array" <- w109
      "Vds array" <- w108
      "corrected PD current array" <- w94
      "Ids array 2" <- w92
      "Corrected PD current array 2" <- w91
      "Vds array 2" <- w90
      "Vgs array 2" <- w89
      "Igs array 2" <- w88
      "?" <- w87
      n162 = local read "Loop"() -> (w97:bool)
      n163 = case shown="True" w97 {
        tunnel: w96 -> [w114 w118]
        tunnel: [w113 w116] -> w86
        frame False {
          n164 = Increment(x=w114) -> (x+1=w113:sgl)
        }
        frame True {
          n165 = Multiply(x=w118, y=sgl 2.0) -> (x*y=w115:sgl)
          n166 = Increment(x=w115) -> (x+1=w116:sgl)
        }
      }
      "Vds points" <- w86
      n167 = Multiply(x=w84, y=sgl 5.0) -> (x*y=w85:sgl)
      n168 = Initialize Array(0.0 ("element"), 0 ("dimension size")) -> (w80:dbl[])
      n169 = Build Array(w80) -> (w81:T2)
      n170 = Resize Matrix(1:w85, 2:w86, 4:w81) -> (0:→"data matrix":T2)
    }
    frame #4 {
      w311 = 0 items=["Set", "Get"] ("Operation (0: Set)")
      w313 = 1 items=["Current", "Voltage"] ("Source Mode (1: Voltage)")
      w310 = 1 items=["Channel 1", "Channel 2"] ("Channel (0: Channel 1)")
      w314 = 1 items=["Pulse", "DC"] ("Source Shape (1: DC)")
      w319 = 0 items=["Set", "Get"] ("Operation (0: Set)")
      w321 = 1 items=["Current", "Voltage"] ("Source Mode (1: Voltage)")
      w318 = 0 items=["Channel 1", "Channel 2"] ("Channel (0: Channel 1)")
      w322 = 1 items=["Pulse", "DC"] ("Source Shape (1: DC)")
      n171 = local read "Agilent address out"() -> (w302:refnum<visa-resource-name>)
      n172 = local read "error out agilent"() -> (w301:errorcluster)
      n173 = local read "light emission ON/OFF"() -> (w326:bool)
      n174 = case shown="True" w326 {
        frame False {
        }
        frame True {
          # "Turn 6487  off"
          n175 = local read "keithley address out"() -> (w328:refnum<k15>)
          n176 = local read "error out keithley"() -> (w327:errorcluster)
          n177 = call <instrlib>:"KE6485 Close.vi"("error in (no error)"=w327, "instrument handle"=w328) -> ("error out"=w329:errorcluster)  [unwired: 9 out]
          n178 = local write "error out keithley"(w329) -> ()
        }
      }
      n179 = call <instrlib>:"Configure Source.vi"("VISA resource name"=w302, "Channel (0: Channel 1)"=w318, "error in (no error)"=w301, "Source Shape (1: DC)"=w322, "Source Mode (1: Voltage)"=w321, "Output Level (0)"=0.0) -> ("VISA resource name out"=w324:refnum<visa-resource-name>, "error out"=w320:errorcluster)  [unwired: 12 in]
      n180 = call <instrlib>:"Enable Output.vi"("Enable Output (T: Enable)"=FALSE, "error in (no error)"=w320, "Operation (0: Set)"=w319, "Channel (0: Channel 1)"=w318, "VISA resource name"=w324) -> ("error out"=w308:errorcluster, "Output Enabled?"=w304:bool, "VISA resource name out"=w309:refnum<visa-resource-name>)  [unwired: 4 in]
      n181 = local write "channel 1 status"(w304) -> ()
      n182 = call <instrlib>:"Configure Source.vi"("VISA resource name"=w309, "Channel (0: Channel 1)"=w310, "error in (no error)"=w308, "Source Shape (1: DC)"=w314, "Source Mode (1: Voltage)"=w313, "Output Level (0)"=0.0) -> ("VISA resource name out"=w316:refnum<visa-resource-name>, "error out"=w312:errorcluster)  [unwired: 12 in]
      n183 = call <instrlib>:"Enable Output.vi"("Enable Output (T: Enable)"=FALSE, "error in (no error)"=w312, "Operation (0: Set)"=w311, "Channel (0: Channel 1)"=w310, "VISA resource name"=w316) -> ("error out"=w307:errorcluster, "Output Enabled?"=w305:bool, "VISA resource name out"=w306:refnum<visa-resource-name>)  [unwired: 4 in]
      n184 = local write "channel 2 status"(w305) -> ()
      n185 = call <instrlib>:"Close.vi"("error in (no error)"=w307, "VISA resource name"=w306) -> ("error out"=w303:errorcluster)  [unwired: 9 in]
      n186 = local write "error out agilent"(w303) -> ()
    }
    frame #5 {
      n187 = local read "corrected PD current array"() -> (w331:dbl[])
      n188 = local read "Vgs array"() -> (w330:dbl[])
      n189 = local read "Vgs array"() -> (w333:dbl[])
      n190 = local read "Ids array"() -> (w334:dbl[])
      n191 = local read "Igs array"() -> (w332:dbl[])
      n192 = Two Button Dialog(message="Do you want to save the data?") -> (T button?=w335:bool)  [unwired: 2 out]
      n193 = case shown="True" w335 {
        tunnel: w333 -> [_ w342]
        tunnel: w334 -> [_ w341]
        tunnel: w332 -> [_ w339]
        tunnel: w331 -> [_ w338]
        tunnel: w330 -> [_ w340]
        frame False {
        }
        frame True {
          n194 = Build Array(w340, w341, w342, w339, w338) -> ()  [unwired: 1 out]
          n195 = local read "data matrix"() -> (w337:dbl[][])
          n196 = call-poly <vilib>:"Write To Spreadsheet File.vi"("transpose? (no:F)"=FALSE, "format (%.3f)"="%.4e", "append to file? (new file:F)"=FALSE, "2D data"=w337) -> ()  [unwired: 4 in, 1 out]
        }
      }
    }
  }
